vi "Translate Wheel_Mecanum.vi"(8 "error in (no error)":errorcluster, 9 "new position":cluster{"x":dbl, "y":dbl}, 10 "wheel index":i32, 11 "mecanum steering frame in":refnum<class "NI_Robotics_Mecanum Steering Frame.lvclass">) -> (0 "error out":errorcluster, 3 "mecanum steering frame out":refnum<class "NI_Robotics_Mecanum Steering Frame.lvclass">)   [LabVIEW 2017, in "NI_Robotics_Configure Steering Frame.lvlib"]
uses:
  <vilib>/robotics/Dialog/Configure Steering Frame/NI_Robotics_Configure Steering Frame.lvlib
  <vilib>/robotics/Steering/Mecanum Steering Frame/NI_Robotics_Mecanum Steering Frame.lvclass
  c:/Program Files (x86)/National Instruments/LabVIEW 2017/vi.lib/robotics/Steering/Steering Frame/NI_Robotics_Steering Frame.lvclass
  <vilib>/robotics/Steering/Steering Frame/NI_Robotics_Steering Frame.lvclass/NI_Robotics_Steering Frame.ctl
  <vilib>/robotics/Steering/Wheel/NI_Robotics_Wheel.lvclass/NI_Robotics_Wheel.ctl
  <vilib>/robotics/Steering/Mecanum Steering Frame/NI_Robotics_Mecanum Steering Frame.lvclass/NI_Robotics_Mecanum Steering Frame.ctl
  <vilib>/robotics/Steering/Mecanum Steering Frame/Wheel Separation to Frame Positions.vi
  <vilib>/robotics/Steering/Steering Frame/Reposition Wheels.vi
  <vilib>/robotics/Steering/Wheel/Update Steering to Wheel Frame Transform.vi
  <vilib>/Analysis/coordinate.llb/Wrap Angle.vi
  <vilib>/Analysis/coordinate.llb/Wrap Angle (scalar).vi
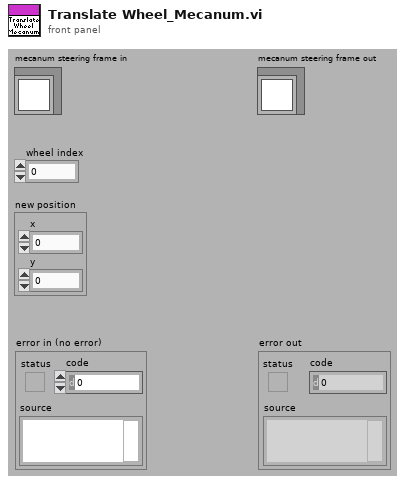
[diagram p1: front panel]
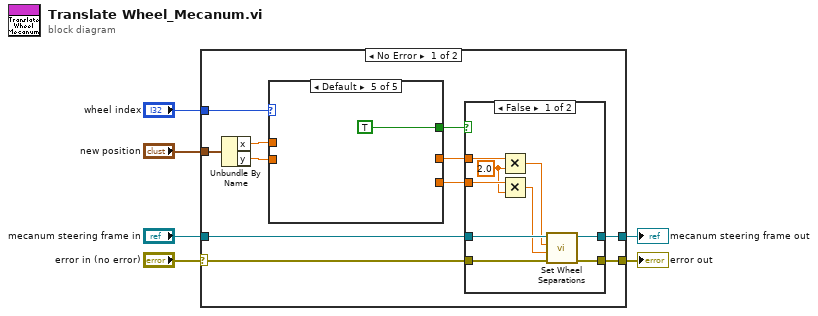
[diagram p0: block diagram]
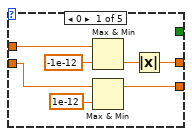
[diagram p3: hidden frame]
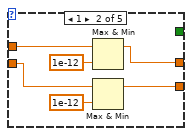
[diagram p4: hidden frame]
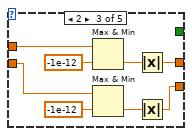
[diagram p5: hidden frame]
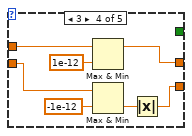
[diagram p6: hidden frame]
diagram:
  n1 = case shown="No Error" "error in (no error)" {
    selector: "error in (no error)" -> [w8 w58]
    tunnel: "mecanum steering frame in" -> [w7 w59]
    tunnel: [w13 w59] -> w4
    tunnel: [w12 w58] -> w3
    tunnel: "wheel index" -> [w17 _]
    tunnel: "new position" -> [w16 _]
    frame No Error {
      n2 = Unbundle By Name(w16) -> ("x"=w15:dbl, "y"=w14:dbl)
      n3 = case shown="Default" w17 {
        tunnel: w15 -> [w35 w41 w49 w56 _]
        tunnel: [w32 w40 w48 w54 _] -> w10
        tunnel: [_ _ _ _ TRUE] -> w11
        tunnel: w14 -> [w31 w37 w43 w52 _]
        tunnel: [w29 w36 w42 w50 _] -> w9
        frame 0 {
          n4 = Max & Min(x=w35, y=-1e-12) -> (min(x,y)=w33:dbl)  [unwired: 1 out]
          n5 = Max & Min(x=w31, y=1e-12) -> (max(x,y)=w29:dbl)  [unwired: 1 out]
          n6 = Absolute Value(x=w33) -> (abs(x)=w32:dbl)
        }
        frame 1 {
          n7 = Max & Min(x=w41, y=1e-12) -> (max(x,y)=w40:dbl)  [unwired: 1 out]
          n8 = Max & Min(x=w37, y=1e-12) -> (max(x,y)=w36:dbl)  [unwired: 1 out]
        }
        frame 2 {
          n9 = Max & Min(x=w49, y=-1e-12) -> (min(x,y)=w47:dbl)  [unwired: 1 out]
          n10 = Max & Min(x=w43, y=-1e-12) -> (min(x,y)=w46:dbl)  [unwired: 1 out]
          n11 = Absolute Value(x=w47) -> (abs(x)=w48:dbl)
          n12 = Absolute Value(x=w46) -> (abs(x)=w42:dbl)
        }
        frame 3 {
          n13 = Max & Min(x=w56, y=1e-12) -> (max(x,y)=w54:dbl)  [unwired: 1 out]
          n14 = Max & Min(x=w52, y=-1e-12) -> (min(x,y)=w51:dbl)  [unwired: 1 out]
          n15 = Absolute Value(x=w51) -> (abs(x)=w50:dbl)
        }
        frame Default {
        }
      }
      n16 = case shown="False" w11 {
        tunnel: w8 -> [w19 w27]
        tunnel: w7 -> [w24 w28]
        tunnel: [w25 w28] -> w13
        tunnel: [w18 w27] -> w12
        tunnel: w10 -> [w26 _]
        tunnel: w9 -> [w22 _]
        frame False {
          w21 = 2.0 ("y")
          n17 = Multiply(x=w26, y=w21) -> (x*y=w23:dbl)
          n18 = Multiply(x=w22, y=w21) -> (x*y=w20:dbl)
          n19 = call <vilib>:"Set Wheel Separations.vi"("error in (no error)"=w19, "wheel separation length"=w20, "wheel separation width"=w23, "mecanum steering frame in"=w24) -> ("error out"=w18:errorcluster, "mecanum steering frame out"=w25:refnum<class "NI_Robotics_Mecanum Steering Frame.lvclass">)  [unwired: 6 in]
        }
        frame True {
        }
      }
    }
    frame Error {
    }
  }
  "mecanum steering frame out" <- w4
  "error out" <- w3
